vi "Filter Name Update the Selector.vi"(8 "error in (no error)":errorcluster, 11 "Post Analysis in":refnum<class "Post Analysis.lvclass">) -> (0 "error out":errorcluster, 3 "Post Analysis out":refnum<class "Post Analysis.lvclass">)   [LabVIEW 2023, in "Data Analysis.lvlib" / "Post Analysis.lvlib" / "Post Analysis.lvclass"]
uses:
  Post Analysis.lvclass
  Post Analysis.lvclass/Post Analysis.ctl
  <userlib>/_OpenG.lib/array/array.llb/Remove Duplicates from 1D Array (String)__ogtk.vi
  HardwareAbstractionLayer_LVOOP/Database/Database.lvclass
  <userlib>/_OpenG.lib/array/array.llb/openg_array.lvlib
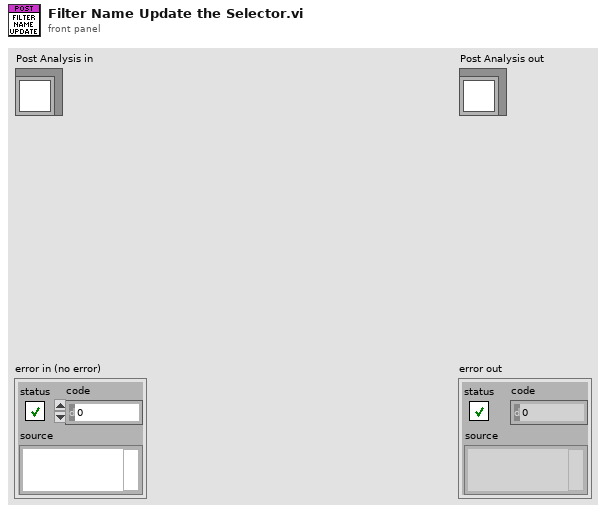
[diagram p1: front panel]
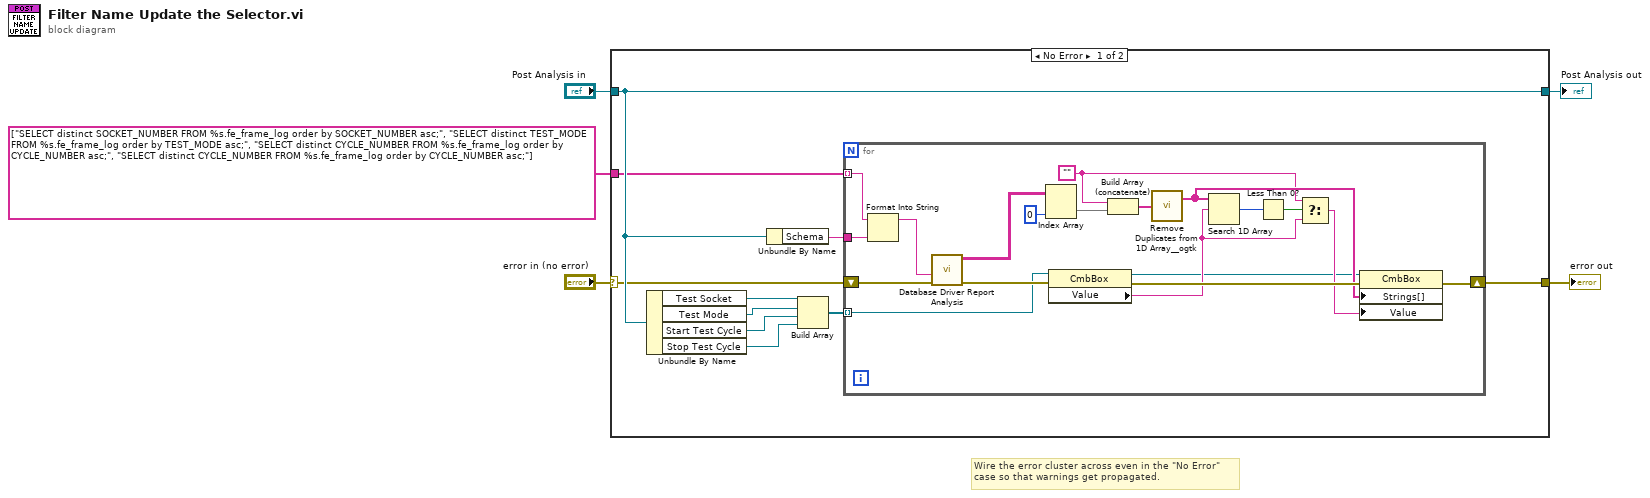
[diagram p0: block diagram]
diagram:
  # "Wire the error cluster across even in the \"No Error\"\ncase so that warnings get propagated."
  n1 = case shown="No Error" "error in (no error)" {
    selector: "error in (no error)" -> [w8 w36]
    tunnel: [w14 w36] -> w4
    tunnel: [w13 w35] -> w2
    tunnel: "Post Analysis in" -> [w13 w35]
    tunnel: string[] ["SELECT distinct SOCKET_NUMBER FROM %s.fe_frame_log order by SOCKET_NUMBER asc;", "SELECT distinct TEST_MODE FROM %s.fe_frame_log order by TEST_MODE asc;", "SELECT distinct CYCLE_NUMBER FROM %s.fe_frame_log order by CYCLE_NUMBER asc;", "SELECT distinct CYCLE_NUMBER FROM %s.fe_frame_log order by CYCLE_NUMBER asc;"] -> [w6 _]
    frame No Error {
      n2 = Unbundle By Name(w13) -> ("Test Socket"=w12:refnum<vi>, "Test Mode"=w11:refnum<vi>, "Start Test Cycle"=w10:refnum<vi>, "Stop Test Cycle"=w9:refnum<vi>)
      n3 = Unbundle By Name(w13) -> ("Schema"=w15:string)
      n4 = Build Array(w12, w11, w10, w9) -> (w7:refnum<vi>[])
      n5 = for {
        shift-right: [w23] -> w14
        shift-left: w8 -> [w34]
        tunnel: w6 -> [w33] mode=indexing
        tunnel: w15 -> [w32]
        tunnel: w7 -> [w25] mode=indexing
        w17 = ""
        n6 = Format Into String(format string=w33, w32) -> (resulting string=w31:string)  [unwired: 2 in, 1 out]
        n7 = call "Database Driver Report Analysis.vi"("error in"=w34, "SQL query"=w31) -> ("error out"=w26:errorcluster, "data"=w30:string[][])  [unwired: 6 in, 2 out]
        n8 = Index Array(array=w30, index (col)=0 ("index (row)")) -> (element=w28:string[])  [unwired: 1 in]
        n9 = property class="CmbBox"(reference=w25, error in=w26) -> (reference out=w16:refnum<vi>, error out=w24:errorcluster, "Value"=w20:string)
        n10 = Build Array (concatenate)(w17, w28) -> (w27:string[])
        n11 = call-poly <userlib>:"Remove Duplicates from 1D Array__ogtk.vi"("Input Array"=w27) -> ("Output Array"=w18:string[])  [unwired: 1 out]
        n12 = Search 1D Array(1D array=w18, element=w20) -> (index of element=w21:i32)  [unwired: 1 in]
        n13 = Less Than 0?(x=w21) -> (x < 0?=w22:bool)
        n14 = Select(t=w17, s=w22, f=w20) -> (s? t:f=w19:string)
        n15 = property class="CmbBox"(reference=w16, error in=w24, "Strings[]"=w18, "Value"=w19) -> (error out=w23:errorcluster)  [unwired: 1 out]
      }
    }
    frame Error {
    }
  }
  "error out" <- w4
  "Post Analysis out" <- w2
